vi "peak detector.vi"(9 "data index":u16, 10 "output valid in":bool, 11 "fft_output":u64) -> (0 "output valid":bool, 1 "adress":u16, 2 "amplitude":u32, 3 "peak":bool)   [LabVIEW 2021]
uses:
  <vilib>/rvi/FXPMathLib/FxpRectToPolar/subVIs/nifxpmath_RectToPolar_SimConfig.ctl
  <vilib>/rvi/FXPMathLib/FxpRectToPolar/simVIs/DllFxpRectToPolarTemp_sub.vi
  <vilib>/rvi/Memory/Memory_Emulation/nirvimemoryFastEmulation.vi
  <vilib>/rvi/Memory/Memory_Emulation/nirvimemoryEmulation.vi
  <vilib>/rvi/Emulation/niFpgaEmulationIsFPGAContextNoSignature.vi
  <vilib>/rvi/DataTransferAndStorage/Container/Common/niFpgaContainerGetUniqueNameForEmu.vi
  <vilib>/rvi/Emulation/niFpgaProcessEmulError.vi
  <vilib>/rvi/Emulation/niFpgaSctlEmulationGetInTimedLoop.vi
  <vilib>/rvi/errors/nirviReportUnexpectedCaseInternalError (U32).vi
  <vilib>/rvi/FXPMathLib/FxpRectToPolar/XNode/nifxpmath_RectToPolar.xnode
  <vilib>/rvi/DataTransferAndStorage/Container/XNode/niFpgaContainer.xnode
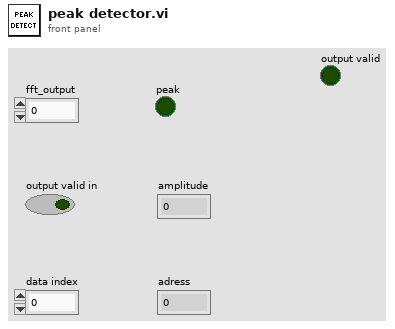
[diagram p1: front panel]
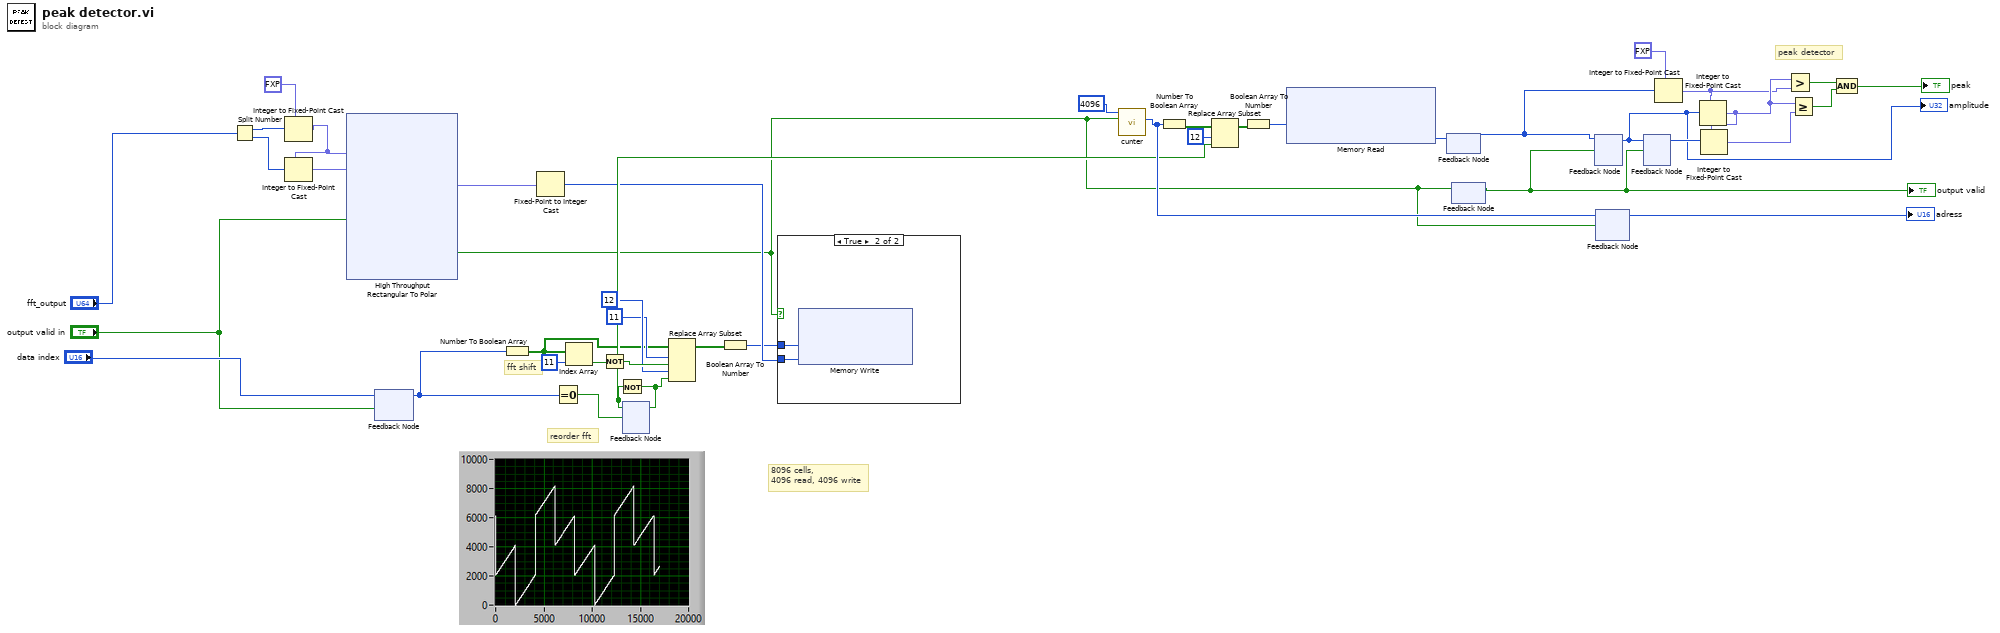
[diagram p0: block diagram]
diagram:
  # "8096 cells,\n4096 read, 4096 write"
  # "reorder fft"
  # "peak detector"
  # "fft shift"
  n1 = Split Number(x="fft_output") -> (hi(x)=w14:u32, lo(x)=w15:u32)
  n2 = Integer to Fixed-Point Cast(fixed-point type=fxp<+/-,32,31> 0.0 ("I"), integer=w14) -> (fixed-point=w17:fxp<+/-,32,31>)
  n3 = Integer to Fixed-Point Cast(fixed-point type=w17, integer=w15) -> (fixed-point=w16:fxp<+/-,32,31>)
  n4 = xnode "High Throughput Rectangular To Polar"("x"=w17, "y"=w16, "input valid"="output valid in") -> ("magnitude"=w31:fxp<+,32,31>, "output valid"=w1:bool)  [unwired: 1 in, 2 out]
  n5 = feedback #1() -> (w29:u16)  [unwired: 1 in]
  n6 = feedback-in #1("data index", "output valid in") -> ()
  n7 = Number To Boolean Array(number=w29) -> (Boolean array=w20:bool[])
  n8 = Fixed-Point to Integer Cast(1:w31) -> (0:w32:u32)
  n9 = Equal To 0?(x=w29) -> (x = 0?=w24:bool)
  n10 = Index Array(array=w20, index=11) -> (element=w19:bool)
  n11 = Not(x=w19) -> (.not. x?=w25:bool)
  n12 = feedback #2() -> (w39:bool)  [unwired: 1 in]
  n13 = Not(x=w39) -> (.not. x?=w26:bool)
  n14 = feedback-in #2(w26, w24) -> ()
  n15 = Replace Array Subset(array=w20, new element #1=w25, index #1=11 ("index"), new element #2=w26, index #2=12 ("index")) -> (w27:bool[])
  n16 = Boolean Array To Number(Boolean array=w27) -> (number=w30:u16)
  n17 = case shown="True" w1 {
    tunnel: w30 -> [_ w44]
    tunnel: w32 -> [_ w43]
    frame False {
    }
    frame True {
      n18 = xnode ("Memory Write")("Address"=w44, "Data"=w43) -> ()  [unwired: 1 in, 1 out]
    }
  }
  n19 = call "cunter.vi"("input valid"=w1, "count to"=u16 4096) -> ("count"=w40:u16)  [unwired: 8 in, 1 out]
  n20 = Number To Boolean Array(number=w40) -> (Boolean array=w34:bool[])
  n21 = Replace Array Subset(array=w34, new element=w39, index=12) -> (w35:bool[])
  n22 = Boolean Array To Number(Boolean array=w35) -> (number=w36:u16)
  n23 = xnode ("Memory Read")("Address"=w36) -> ("Data"=w3:u32)  [unwired: 1 in, 1 out]
  n24 = feedback #3() -> (w4:u32)  [unwired: 1 in]
  n25 = feedback-in #3(w3) -> ()
  n26 = feedback #4() -> (w2:bool)  [unwired: 1 in]
  "output valid" <- w2
  n27 = feedback-in #4(w1) -> ()
  n28 = feedback #5() -> (w5:u32)  [unwired: 1 in]
  "amplitude" <- w5
  n29 = feedback-in #5(w4, w2) -> ()
  n30 = feedback #6() -> (→"adress":u16)  [unwired: 1 in]
  n31 = feedback-in #6(w40, w1) -> ()
  n32 = feedback #7() -> (w9:u32)  [unwired: 1 in]
  n33 = feedback-in #7(w5, w2) -> ()
  n34 = Integer to Fixed-Point Cast(fixed-point type=fxp<+,32,31> 0.0 ("magnitude"), integer=w4) -> (fixed-point=w6:fxp<+,32,31>)
  n35 = Integer to Fixed-Point Cast(fixed-point type=w6, integer=w5) -> (fixed-point=w7:fxp<+,32,31>)
  n36 = Integer to Fixed-Point Cast(fixed-point type=w7, integer=w9) -> (fixed-point=w8:fxp<+,32,31>)
  n37 = Greater?(x=w7, y=w6) -> (0:w11:bool)
  n38 = Greater Or Equal?(x=w7, y=w8) -> (x >= y?=w38:bool)
  n39 = Compound Arithmetic op=AND(w11, w38) -> (→"peak":bool)
